vi "Reconnect.vi"(8 "error in (no error)":errorcluster, 11 "UDP Reader in":refnum<class "UDP Reader.lvclass">) -> (0 "error out":errorcluster, 3 "UDP Reader out":refnum<class "UDP Reader.lvclass">)   [LabVIEW 2022 SP3, in "UDP Reader.lvlib" / "UDP Reader.lvclass"]
uses:
  UDP Reader.lvclass
  UDP Reader.lvclass/UDP Reader.ctl
  <vilib>/Utility/tcp.llb/UDP Multicast Read-Only Open.vi
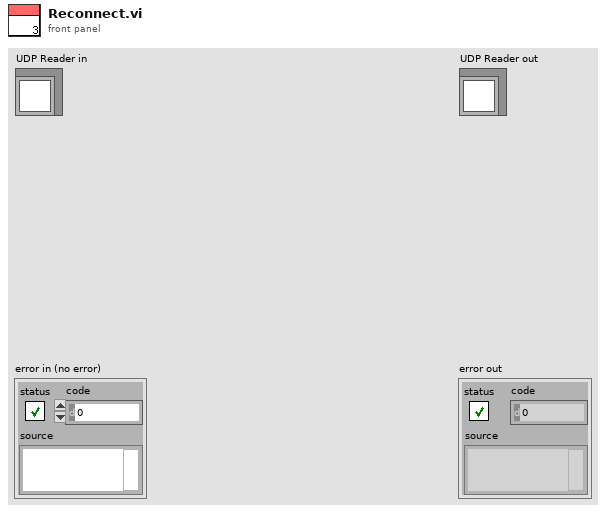
[diagram p1: front panel]
types:
  T1 = typedef "UDP Input.ctl" = cluster{"Local IP":string, "Port":string, "Server IP":string}
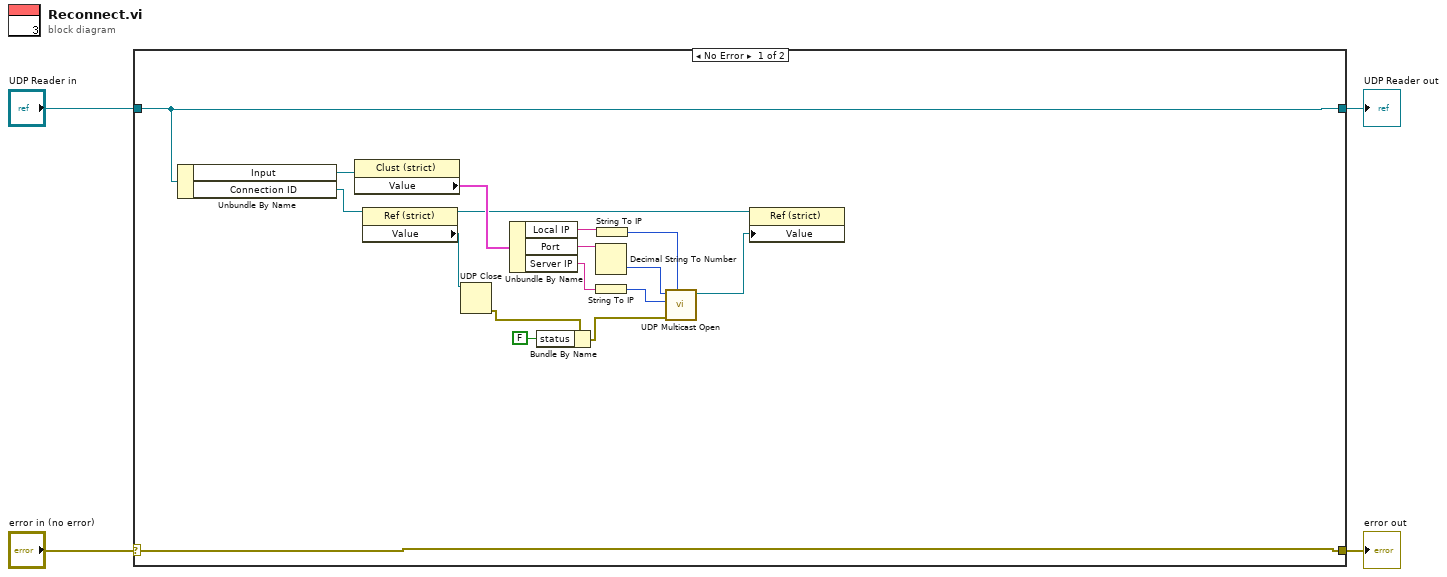
[diagram p0: block diagram]
diagram:
  n1 = case shown="No Error" "error in (no error)" {
    selector: "error in (no error)" -> [w9 w23]
    tunnel: [w9 w23] -> w3
    tunnel: [w11 w22] -> w1
    tunnel: "UDP Reader in" -> [w11 w22]
    frame No Error {
      n2 = Unbundle By Name(w11) -> ("Input"=w18:refnum<vi>, "Connection ID"=w13:refnum<vi>)
      n3 = property class="Clust (strict)"(reference=w18) -> ("Value"=w17:T1)  [unwired: 1 in, 2 out]
      n4 = property class="Ref (strict)"(reference=w13) -> (reference out=w5:refnum<vi>, "Value"=w12:refnum<k16>)  [unwired: 1 in, 1 out]
      n5 = UDP Close(connection ID=w12) -> (error out=w8:errorcluster)  [unwired: 1 in, 1 out]
      n6 = Unbundle By Name(w17) -> ("Local IP"=w16:string, "Port"=w15:string, "Server IP"=w14:string)
      n7 = Bundle By Name(cluster=w8, "status"=FALSE) -> (w7:errorcluster)
      n8 = Decimal String To Number(string=w15) -> (number=w20:i32)  [unwired: 2 in, 1 out]
      n9 = String To IP(1:w14) -> (0:w21:u32)
      n10 = String To IP(1:w16) -> (0:w19:u32)
      n11 = call-poly <vilib>:"UDP Multicast Open.vi"("net address"=w19, "error in (no error)"=w7, "multicast addr"=w21, "port"=w20) -> ("connection ID"=w6:refnum<k16>)  [unwired: 5 in, 2 out]
      n12 = property class="Ref (strict)"(reference=w5, "Value"=w6) -> ()  [unwired: 1 in, 2 out]
    }
    frame Error {
    }
  }
  "error out" <- w3
  "UDP Reader out" <- w1
